vi "Deserialise metadata.vi"(8 "error in (no error)":errorcluster, 10 "JSON String to decode":string, 11 "object in":refnum<class "Message Class.lvclass">) -> (0 "error out":errorcluster, 3 "object out":refnum<class "Message Class.lvclass">)   [LabVIEW 2018, in "ClientMessaging.lvlib" / "Message Class.lvclass"]
doc: "Deserialise a string with metadata"
uses:
  Message Class.lvclass
  Message Class.lvclass/Message Class.ctl
  <vilib>/addons/_JKI.lib/Serialization/JSON/JKI JSON Serialization.lvlib
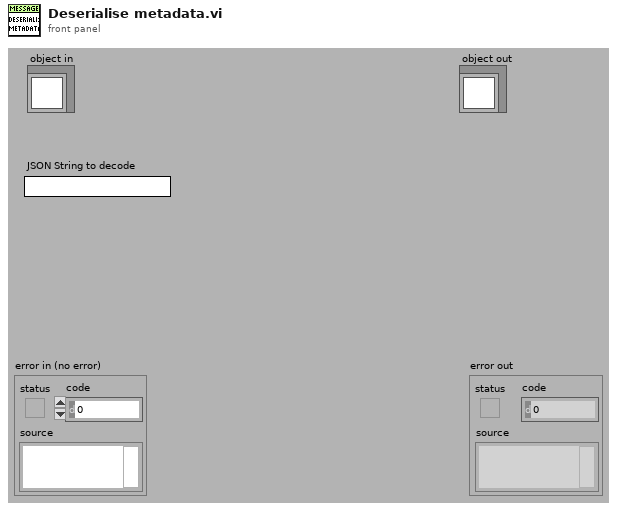
[diagram p1: front panel]
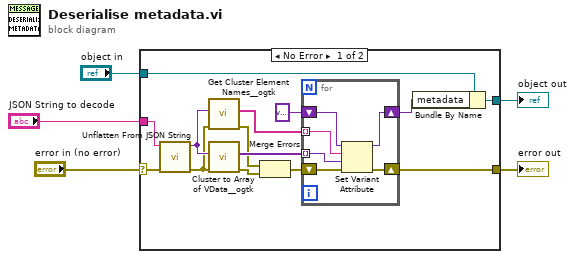
[diagram p0: block diagram]
diagram:
  n1 = case shown="No Error" "error in (no error)" {
    selector: "error in (no error)" -> [w9 w27]
    tunnel: [w8 w27] -> w2
    tunnel: [w18 w26] -> w1
    tunnel: "object in" -> [w19 w26]
    tunnel: "JSON String to decode" -> [w17 _]
    frame No Error {
      n2 = call <vilib>:"Unflatten From JSON String.vi"("error in (no error)"=w9, "JSON String"=w17) -> ("error out"=w11:errorcluster, "Variant"=w16:variant)  [unwired: 8 in]
      n3 = call <userlib>:"Get Cluster Element Names__ogtk.vi"("error in (no error)"=w11, "Cluster"=w16) -> ("error out"=w10:errorcluster, "Element Names"=w14:string[])  [unwired: 8 in]
      n4 = call <userlib>:"Cluster to Array of VData__ogtk.vi"("error in (no error)"=w11, "Cluster"=w16) -> ("error out"=w6:errorcluster, "Array of VData"=w13:variant[])  [unwired: 8 in]
      n5 = Merge Errors(w10, w6) -> (w7:errorcluster)
      n6 = for {
        shift-right: [w22] -> w12
        shift-left: variant -> [w25]
        tunnel: w14 -> [w24] mode=indexing
        tunnel: w13 -> [w23] mode=indexing
        shift-right: [w20] -> w8
        shift-left: w7 -> [w21]
        n7 = Set Variant Attribute(Variant=w25, name=w24, value=w23, error in=w21) -> (Variant out=w22:variant, error out=w20:errorcluster)  [unwired: 1 out]
      }
      n8 = Bundle By Name(cluster=w19, "metadata"=w12) -> (w18:refnum<class "Message Class.lvclass">)
    }
    frame Error {
    }
  }
  "error out" <- w2
  "object out" <- w1
